vi "ExcelClose.vi"(8 "error":errorcluster caption="错误输入（无错误）", 11 "Excel.Open":refnum<k7>) -> (0 "error out":errorcluster caption="错误输出", 3 "Excel.Open":refnum<k7>)   [LabVIEW 2014]
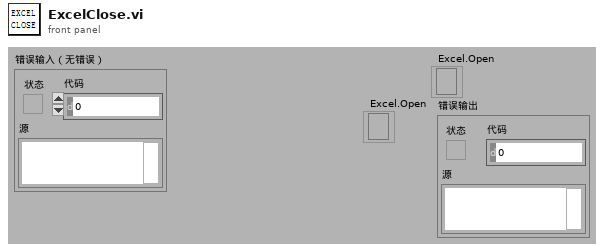
[diagram p1: front panel]
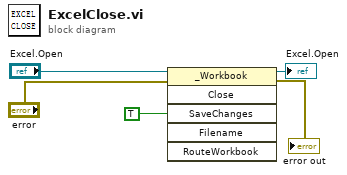
[diagram p0: block diagram]
diagram:
  n1 = invoke class="_Workbook" method="Close"(reference="Excel.Open", error in="error", "SaveChanges"=TRUE) -> (reference out=→"Excel.Open":refnum<k7>, error out=→"error out":errorcluster)  [unwired: 3 in, 4 out]
